vi "fpga.vi"() -> ()   [LabVIEW 2014]
uses:
  <vilib>/rvi/Emulation/niFpgaGetClockAttributes.vi
  <vilib>/rvi/Emulation/niFpgaSctlEmulationGetInTimedLoop.vi
  <vilib>/rvi/Emulation/niFpgaEmulationReportErrorSimple.vi
  <vilib>/rvi/eio/common/nirviEmuTemplateMethod_errors.vi
  <vilib>/rvi/Emulation/niFpgaCriticalErrorInLSC.vi
  <vilib>/eio/EIONode/EIONode.xnode
panel:
  in  "AO0":fxp<+/-,20,5>
  out "AI0":fxp<+/-,24,5>
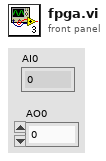
[diagram p1: front panel]
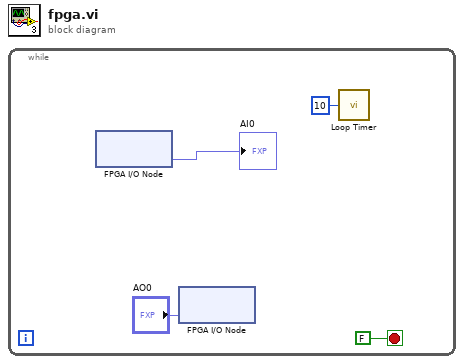
[diagram p0: block diagram]
diagram:
  n1 = while {
    stop <- FALSE stop-if-true
    n2 = xnode "FPGA I/O Node"() -> ("AI0"=→"AI0":fxp<+/-,24,5>)  [unwired: 1 in, 1 out]
    n3 = xnode "FPGA I/O Node"("AO0"="AO0") -> ()  [unwired: 1 in, 1 out]
    n4 = call "Loop Timer"("Count(Ticks)"=u32 10) -> ()  [unwired: 1 out]
  }
